vi "Get Used Path Tags.vi"(8 "error in (no error)":errorcluster, 11 "Log File Specification in":refnum<class "Log File Specification.lvclass">) -> (0 "error out":errorcluster, 2 "Used Path Tags":string[](array[string]), 3 "Log File Specification out":refnum<class "Log File Specification.lvclass">)   [LabVIEW 2015, in "Waveform Data Logger Shared.lvlib" / "Log File Specification.lvclass"]
doc: "Returns the list of tags used in the base file path."
uses:
  Log File Specification.lvclass
  Log File Specification.lvclass/Log File Specification.ctl
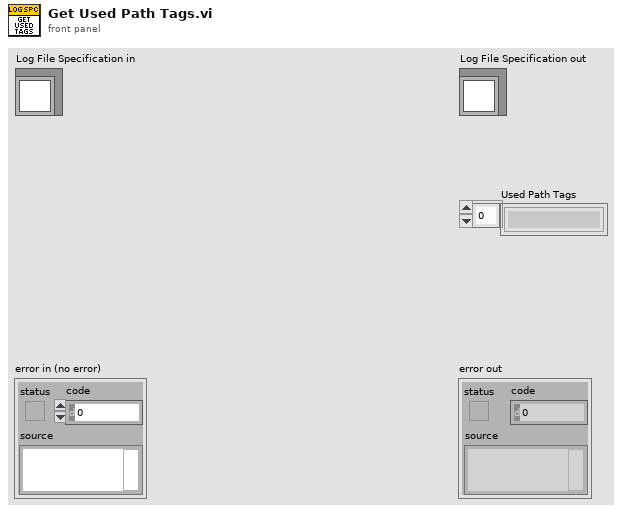
[diagram p1: front panel]
types:
  T1 = typedef "Waveform Data Logger Shared.lvlib/Log File Specification.lvclass/Path Segment.ctl" = cluster{"String":string, "Is Tag":bool}
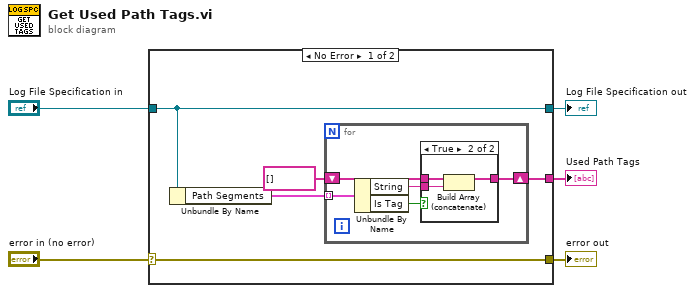
[diagram p0: block diagram]
diagram:
  n1 = case shown="No Error" "error in (no error)" {
    selector: "error in (no error)" -> [w10 w21]
    tunnel: [w10 w21] -> w4
    tunnel: [w9 w20] -> w2
    tunnel: "Log File Specification in" -> [w9 w20]
    tunnel: [w6 _] -> w1
    frame No Error {
      n2 = Unbundle By Name(w9) -> ("Path Segments"=w8:T1[])
      n3 = for {
        tunnel: w8 -> [w15] mode=indexing
        shift-right: [w12] -> w6
        shift-left: string[] [] -> [w11]
        n4 = Unbundle By Name(w15) -> ("String"=w13:string, "Is Tag"=w14:bool)
        n5 = case shown="True" w14 {
          tunnel: w13 -> [_ w19]
          tunnel: [w16 w18] -> w12
          tunnel: w11 -> [w16 w17]
          frame False {
          }
          frame True {
            n6 = Build Array (concatenate)(w17, w19) -> (w18:string[])
          }
        }
      }
    }
    frame Error {
    }
  }
  "error out" <- w4
  "Log File Specification out" <- w2
  "Used Path Tags" <- w1
